vi "Temperature Conversion.vi"(9 "Calibration Array":T1, 11 "Raw ADC Array":dbl[](array[numeric])) -> (3 "Temperature Array":dbl[](array[numeric]))   [LabVIEW 2021]
uses:
  Controls/Temperature Calibration Array.ctl
  Controls/Temperature Calibration.ctl
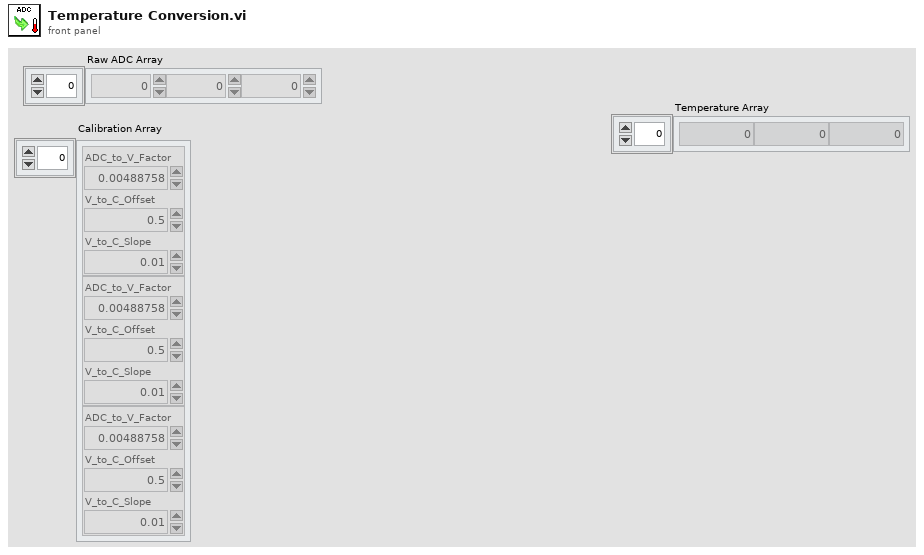
[diagram p1: front panel]
types:
  T1 = typedef "Temperature Calibration Array.ctl" = T2[]
  T2 = typedef "Temperature Calibration.ctl" = cluster{"ADC_to_V_Factor":dbl, "V_to_C_Offset":dbl, "V_to_C_Slope":dbl}
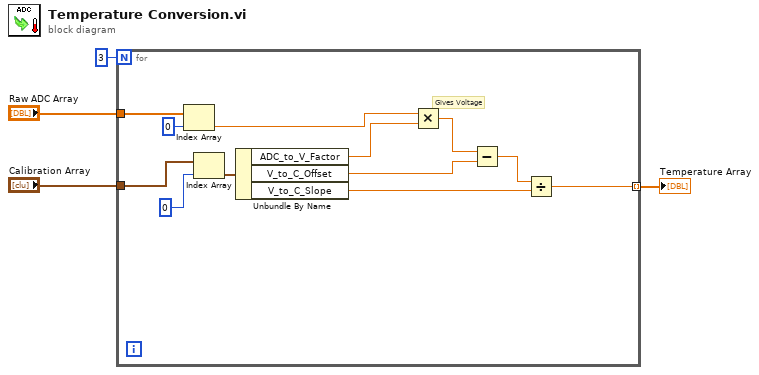
[diagram p0: block diagram]
diagram:
  n1 = for {
    N: 3 -> [_]
    tunnel: "Raw ADC Array" -> [w7]
    tunnel: "Calibration Array" -> [w16]
    tunnel: [w9] -> w3 mode=indexing
    # "Gives Voltage"
    n2 = Index Array(array=w7, index=0) -> (element=w6:dbl)
    n3 = Index Array(array=w16, index=0) -> (element=w15:T2)
    n4 = Unbundle By Name(w15) -> ("ADC_to_V_Factor"=w14:dbl, "V_to_C_Offset"=w12:dbl, "V_to_C_Slope"=w10:dbl)
    n5 = Multiply(x=w6, y=w14) -> (x*y=w13:dbl)
    n6 = Subtract(x=w13, y=w12) -> (x-y=w11:dbl)
    n7 = Divide(x=w11, y=w10) -> (x/y=w9:dbl)
  }
  "Temperature Array" <- w3
